vi "Gravity_Calculation.vi"(8 "Current Linear Speed":dbl, 9 "Array prev":dbl[](array[numeric]), 10 "Current Linear Speed prev":dbl) -> (2 "Array":dbl[](array[numeric]), 3 "Acceleration due to gravity":dbl)   [LabVIEW 2018]
doc: "This VI calculates the average value of acceleration due to gravity of a falling object. It does so by calculating the change in linear speed by subtracting previous linear speed from current linear speed. It then calculates current linear acceleration and then dividing it by change in time (0.1 s). If the calculated value falls within +/- 10 % error of 9.81 (average accepted value for acceleration due to gravity) then it is added to an array of acceleration values and divided by the number of elements in that array to calculate the average value of acceleration due to gravity.\n\nInputs:\nCurrent linear speed prev;\nArray prev;\nCurrent linear speed.\n\nOutputs:\nAcceleration due to gravity;\nArray."
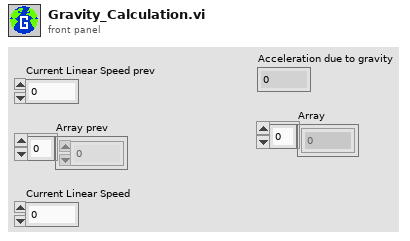
[diagram p1: front panel]
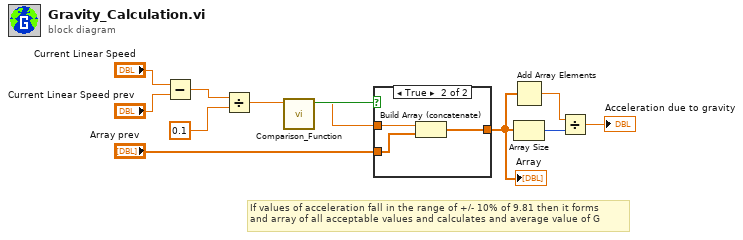
[diagram p0: block diagram]
diagram:
  # "If values of acceleration fall in the range of +/- 10% of 9.81 then it forms\nand array of all acceptable values and calculates and average value of G"
  n1 = Subtract(x="Current Linear Speed", y="Current Linear Speed prev") -> (x-y=w10:dbl)
  n2 = Divide(x=w10, y=0.1) -> (x/y=w6:dbl)
  n3 = call "Comparison_Function.vi"("Value of acceleration due to gravity"=w6) -> ("Within Specified Value?"=w7:bool)  [unwired: 10 in]
  n4 = case shown="True" w7 {
    tunnel: w6 -> [_ w15]
    tunnel: [w12 w14] -> w3
    tunnel: "Array prev" -> [w12 w13]
    frame False {
    }
    frame True {
      n5 = Build Array (concatenate)(w15, w13) -> (w14:dbl[])
    }
  }
  "Array" <- w3
  n6 = Add Array Elements(numeric array=w3) -> (sum=w4:dbl)
  n7 = Array Size(array=w3) -> (size(s)=w2:i32)
  n8 = Divide(x=w4, y=w2) -> (x/y=→"Acceleration due to gravity":dbl)
